vi "_RT_CtrlLoop_Log initProfile.vi"(8 "error in (no error)":errorcluster) -> (0 "error out":errorcluster, 2 "all rows":string[][](array[string]), 3 "new file path":path)   [LabVIEW 2018]
uses:
  <vilib>/Utility/file.llb/Read Delimited Spreadsheet (string).vi
  <vilib>/Utility/file.llb/Write Delimited Spreadsheet (string).vi
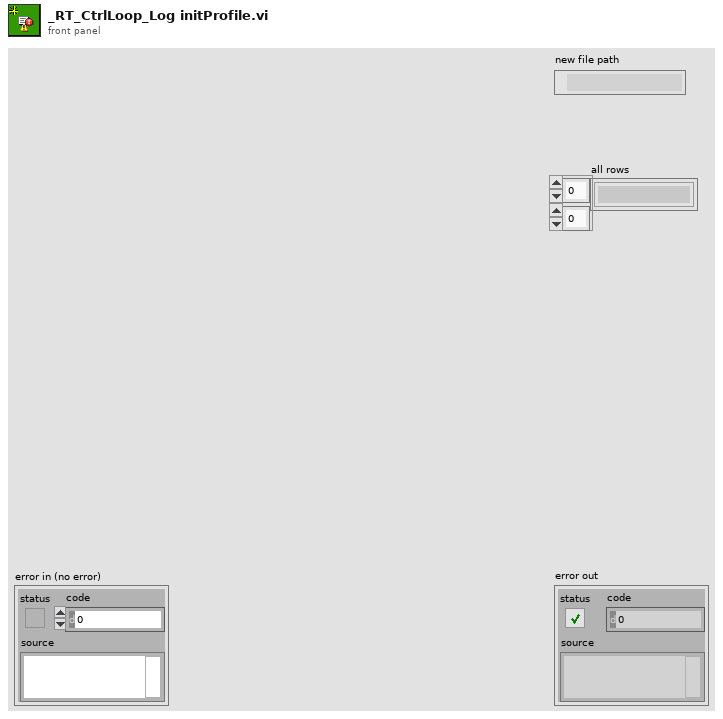
[diagram p1: front panel]
types:
  T1 = enum16{"open", "replace", "create", "open or create", "replace or create", "replace or create with confirmation"}
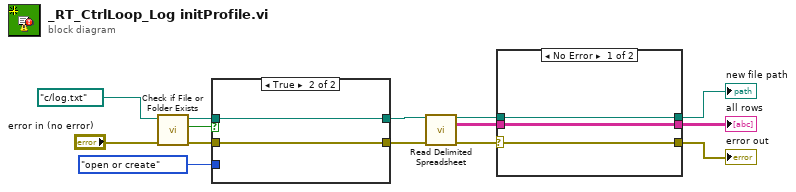
[diagram p0: block diagram]
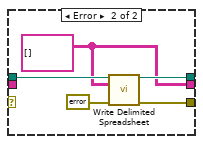
[diagram p2: hidden frame]
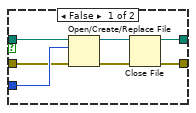
[diagram p3: hidden frame]
diagram:
  n1 = call <vilib>:"Check if File or Folder Exists.vi"("error in (no error)"="error in (no error)", "path"=path "c:/log.txt") -> ("error out"=w12:errorcluster, "file or folder exists?"=w14:bool, "dup path"=w13:path)  [unwired: 7 in]
  n2 = case shown="True" w14 {
    tunnel: w13 -> [w19 w23]
    tunnel: w12 -> [w17 w22]
    tunnel: T1."open or create" ("operation (0:open)") -> [w18 _]
    tunnel: [w16 w23] -> w10
    tunnel: [w15 w22] -> w9
    frame False {
      n3 = Open/Create/Replace File(file path (use dialog)=w19, error in=w17, operation (0:open)=w18) -> (refnum out=w21:refnum<file>, error out=w20:errorcluster)  [unwired: 3 in, 1 out]
      n4 = Close File(refnum=w21, error in=w20) -> (path=w16:path, error out=w15:errorcluster)
    }
    frame True {
    }
  }
  n5 = call-poly <vilib>:"Read Delimited Spreadsheet.vi"("file path (dialog if empty)"=w10, "error in (no error)"=w9) -> ("new file path (Not A Path if cancelled)"=w6:path, "all rows"=w5:string[][], "error out"=w4:errorcluster)  [unwired: 8 in, 3 out]
  n6 = case shown="No Error" w4 {
    selector: w4 -> [w26 _]
    tunnel: [w26 w29] -> w1
    tunnel: w6 -> [w25 w30]
    tunnel: w5 -> [w24 _]
    tunnel: [w25 w28] -> w3
    tunnel: [w24 w27] -> w2
    frame No Error {
    }
    frame Error {
      w27 = string[][] [] ("element")
      n7 = call-poly <vilib>:"Write Delimited Spreadsheet.vi"("file path (dialog if empty)"=w30, "2D data"=w27, "error in (no error)"=errorcluster {"status"=FALSE, "code"=0, "source"=""}) -> ("new file path (Not A Path if cancelled)"=w28:path, "error out"=w29:errorcluster)  [unwired: 11 in]
    }
  }
  "new file path" <- w3
  "error out" <- w1
  "all rows" <- w2
